vi "TestExec.Config, Read ScriptSearchPaths.vi"(8 "error in":errorcluster, 11 "Station Data Dir Config File":path) -> (0 "error out":errorcluster, 3 "ScriptSearchPaths":path[](array[path]))   [LabVIEW 2018]
uses:
  <vilib>/Utility/config.llb/Read Key (Path).vi
  <vilib>/Utility/config.llb/NI_LVConfig.lvlib
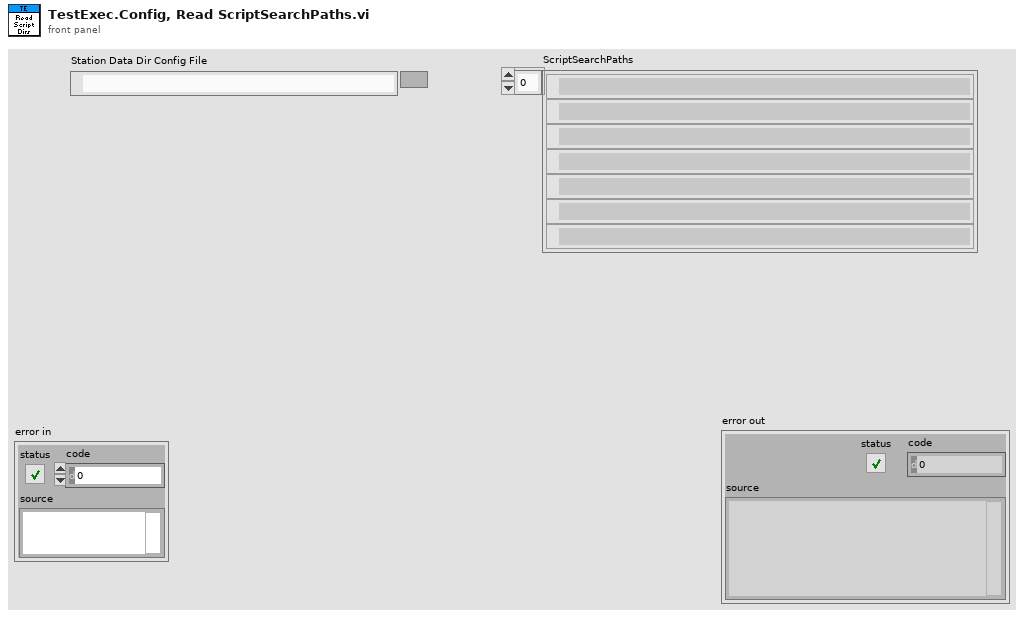
[diagram p1: front panel]
types:
  T1 = typedef "NI_LVConfig.lvlib/Config Data RefNum.ctl" = refnum<k1>
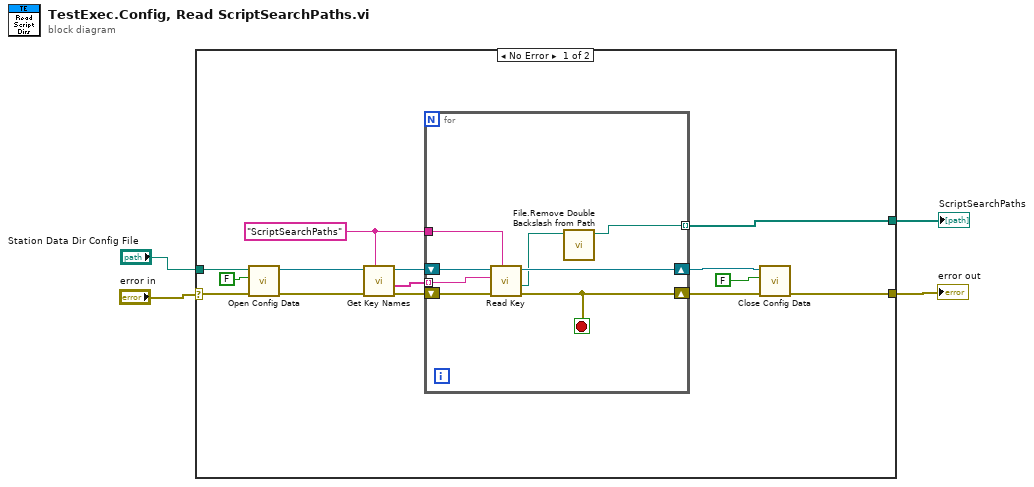
[diagram p0: block diagram]
diagram:
  n1 = case shown="No Error" "error in" {
    selector: "error in" -> [w14 w27]
    tunnel: "Station Data Dir Config File" -> [w18 _]
    tunnel: [w17 w27] -> w3
    tunnel: [w5 _] -> w1
    frame No Error {
      w8 = "ScriptSearchPaths"
      n2 = call <vilib>:"Open Config Data.vi"("error in (no error)"=w14, "create file if necessary (T)"=FALSE, "configuration file path"=w18) -> ("error out"=w12:errorcluster, "refnum"=w13:T1)  [unwired: 6 in, 1 out]
      n3 = call <vilib>:"Get Key Names.vi"("section"=w8, "error in (no error)"=w12, "refnum"=w13) -> ("error out"=w10:errorcluster, "key names"=w9:string[], "refnum out"=w11:T1)  [unwired: 5 in, 1 out]
      n4 = for {
        tunnel: w9 -> [w23] mode=indexing
        tunnel: w8 -> [w24]
        tunnel: [w19] -> w5 mode=indexing
        shift-right: [w21] -> w6
        shift-left: w11 -> [w26]
        shift-right: [w22] -> w7
        shift-left: w10 -> [w25]
        stop <- w22 stop-if-true
        n5 = call-poly <vilib>:"Read Key.vi"("section"=w24, "error in (no error)"=w25, "key"=w23, "refnum"=w26) -> ("error out"=w22:errorcluster, "value"=w20:path, "refnum out"=w21:T1)  [unwired: 4 in, 1 out]
        n6 = call "File.Remove Double Backslash from Path.vi"("Path"=w20) -> ("Path Out"=w19:path)  [unwired: 10 in]
      }
      n7 = call <vilib>:"Close Config Data.vi"("error in (no error)"=w7, "write file if changed (T)"=FALSE, "refnum"=w6) -> ("error out"=w17:errorcluster)  [unwired: 7 in, 1 out]
    }
    frame Error {
    }
  }
  "error out" <- w3
  "ScriptSearchPaths" <- w1
